vi "subscribe.vi"(10 "type":string="std_msgs/String", 11 "topic":string="/chatter") -> (3 "JSON字符串":string)   [LabVIEW 2014]
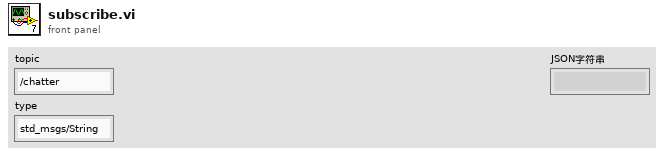
[diagram p1: front panel]
types:
  T1 = cluster{"op":string, "topic":string, "type":string}
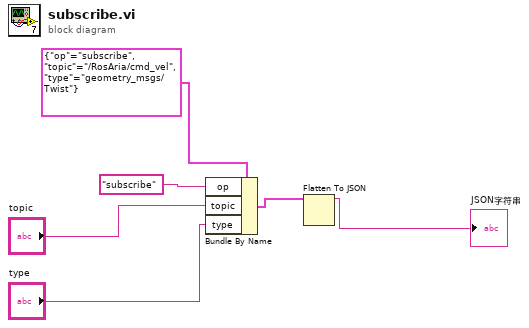
[diagram p0: block diagram]
diagram:
  n1 = Bundle By Name(cluster=T1 {"op"="subscribe", "topic"="/RosAria/cmd_vel", "type"="geometry_msgs/Twist"} ("输出簇"), "op"="subscribe", "topic"="topic", "type"="type") -> (w2:T1)
  n2 = Flatten To JSON(anything=w2) -> (JSON string=→"JSON字符串":string)  [unwired: 2 in, 1 out]
